vi "Polynomial Roots (CDB).vi"(10 "option":u16(ring) items=["General"=0, "Advanced Refinement"=3], 11 "P(x)":cdb[](array[numeric]) format="%#.6g") -> (0 "error":i32, 3 "Roots":cdb[](array[numeric]) format="%#.6g")   [LabVIEW 2018, in "NI_AALPro.lvlib"]
doc: "Finds the roots of polynomial <B>P(x)</B>. This VI removes leading coefficients of the polynomial that are equal to zero. Wire data to the <B>P(x)</B> input to determine the polymorphic instance to use or manually select the instance."
uses:
  NI_AALPro.lvlib
  Remove Zero Coefficients (CDB).vi
  <resource>/lvanlys.dll
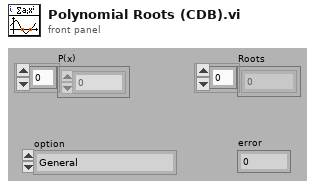
[diagram p1: front panel]
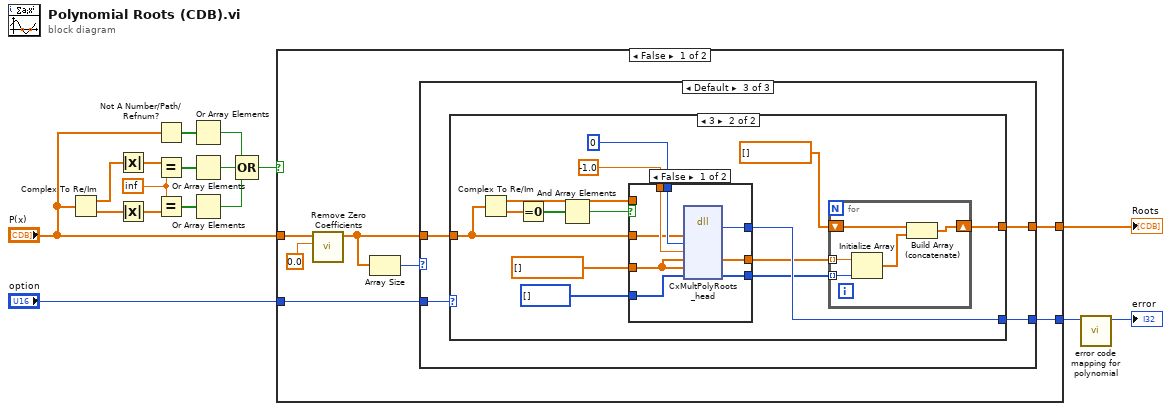
[diagram p0: block diagram]
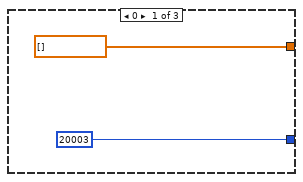
[diagram p2: hidden frame]
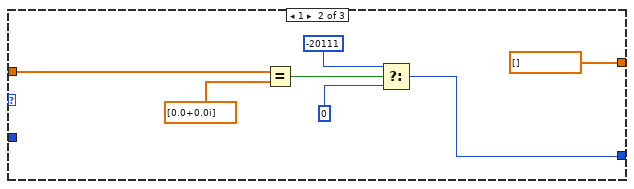
[diagram p3: hidden frame]
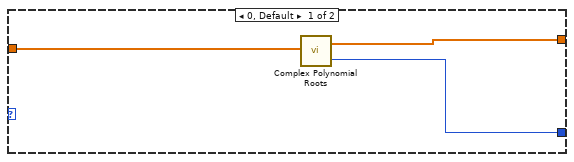
[diagram p4: hidden frame]
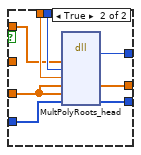
[diagram p5: hidden frame]
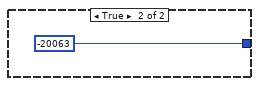
[diagram p6: hidden frame]
diagram:
  w3 = inf
  n1 = Complex To Re/Im(x + iy="P(x)") -> (x=w4:dbl[], y=w7:dbl[])
  n2 = Absolute Value(x=w4) -> (abs(x)=w5:dbl[])
  n3 = Absolute Value(x=w7) -> (abs(x)=w12:dbl[])
  n4 = Not A Number/Path/Refnum?(number/path/refnum="P(x)") -> (NaN/Path/Refnum?=w13:bool[])
  n5 = Equal?(x=w5, y=w3) -> (x = y?=w6:bool[])
  n6 = Equal?(x=w3, y=w12) -> (x = y?=w11:bool[])
  n7 = Or Array Elements(Boolean array=w13) -> (logical OR=w2:bool)
  n8 = Or Array Elements(Boolean array=w6) -> (logical OR=w1:bool)
  n9 = Or Array Elements(Boolean array=w11) -> (logical OR=w10:bool)
  n10 = Compound Arithmetic op=OR(w2, w1, w10) -> (w9:bool)
  n11 = case shown="False" w9 {
    tunnel: [w24 _] -> w17
    tunnel: "option" -> [w22 _]
    tunnel: [w21 -20063 ("error")] -> w15
    tunnel: "P(x)" -> [w19 _]
    frame False {
      n12 = call-poly "Remove Zero Coefficients.vi"("threshold"=0.0, "P(x) In"=w19) -> ("P(x) Out"=w18:cdb[])  [unwired: 1 in, 8 out]
      n13 = Array Size(array=w18) -> (size(s)=w23:i32)
      n14 = case shown="Default" w23 {
        tunnel: [cdb[] [] ("Polynomial Roots") cdb[] [] ("Approximate Roots") w37] -> w24
        tunnel: [20003 ("empty array") w27 w35] -> w21
        tunnel: w18 -> [_ w32 w34]
        tunnel: w22 -> [_ _ w36]
        frame 0 {
        }
        frame 1 {
          n15 = Equal?(x=w32, y=cdb[] [0.0+0.0i]) -> (x = y?=w30:bool)
          n16 = Select(t=-20111, s=w30, f=0) -> (s? t:f=w27:i32)
        }
        frame Default {
          n17 = case shown="3" w36 {
            tunnel: [w39 w53] -> w37
            tunnel: w34 -> [w40 w45]
            tunnel: [w38 w52] -> w35
            frame 0, Default {
              n18 = call "Complex Polynomial Roots.vi"("Polynomial"=w40) -> ("Polynomial Roots"=w39:cdb[], "error"=w38:i32)
            }
            frame 3 {
              n19 = Complex To Re/Im(x + iy=w45) -> (x=w41:dbl[], y=w44:dbl[])
              n20 = Equal To 0?(x=w44) -> (x = 0?=w43:bool[])
              n21 = And Array Elements(Boolean array=w43) -> (logical AND=w42:bool)
              n22 = case shown="False" w42 {
                tunnel: [w62 w65] -> w52
                tunnel: i32[] [] -> [w61 w66]
                tunnel: [w60 w63] -> w50
                tunnel: cdb[] [] ("Roots") -> [w59 w67]
                tunnel: [w58 w64] -> w48
                tunnel: -1.0 ("tol") -> [w57 w69]
                tunnel: 0 ("alg2") -> [w56 w70]
                tunnel: w45 -> [w55 _]
                tunnel: w41 -> [_ w68]
                frame False {
                  n23 = dll-call lib="C:/Program Files (x86)/National Instruments/LabVIEW 2018/resource/lvanlys.*" fn="CxMultPolyRoots_head"("pH"=w55, "alg2"=w56, "tol"=w57, "approotH"=w59, "rootH"=w59, "multH"=w61) -> ("return type"=w62:i32, "approotH"=w58:cdb[], "multH"=w60:i32[])  [unwired: 7 in, 2 out]
                }
                frame True {
                  n24 = dll-call lib="C:/Program Files (x86)/National Instruments/LabVIEW 2018/resource/lvanlys.*" fn="MultPolyRoots_head"("pH"=w68, "alg2"=w70, "tol"=w69, "appRootH"=w67, "rootH"=w67, "multH"=w66) -> ("return type"=w65:i32, "appRootH"=w64:cdb[], "multH"=w63:i32[])  [unwired: 7 in, 2 out]
                }
              }
              n25 = for {
                shift-right: [w71] -> w53
                shift-left: cdb[] [] ("Approximate Roots") -> [w72]
                tunnel: w50 -> [w75] mode=indexing
                tunnel: w48 -> [w74] mode=indexing
                n26 = Initialize Array(w74, w75) -> (w73:cdb[])
                n27 = Build Array (concatenate)(w72, w73) -> (w71:cdb[])
              }
            }
          }
        }
      }
    }
    frame True {
    }
  }
  "Roots" <- w17
  n28 = call "error code mapping for polynomial.vi"("error in"=w15) -> ("error out"=→"error":i32)  [unwired: 10 out]
